vi "Day 13-1.vi"() -> ()   [LabVIEW 2019, in "Day 13.lvlib"]
uses:
  Day 13.lvlib
panel:
  out "size(s)":i32[](array[numeric])
  out "Numeric":i32
  out "Result":bool[][](array[boolean])
  out "Without fold":bool[][](array[boolean])
  out "coordenate":i32[](array[numeric])
  out "axis":string[](array[string])
  out "Points coordenates":i32[][](array[numeric])
  in  "String":string
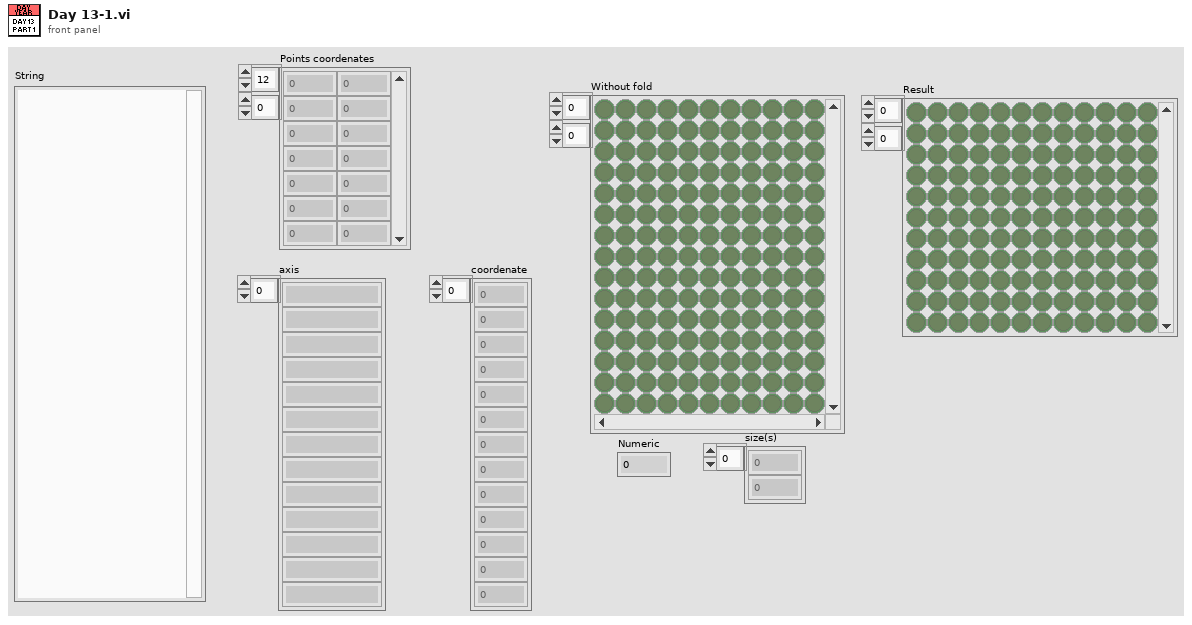
[diagram p1: front panel]
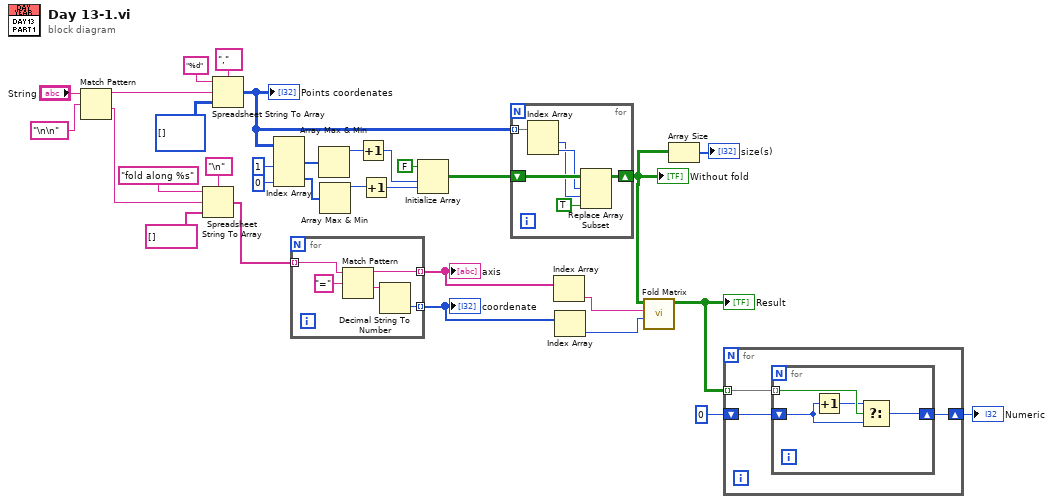
[diagram p0: block diagram]
diagram:
  n1 = Match Pattern(string="String", regular expression="\n\n") -> (before substring=w27:string, after substring=w22:string)  [unwired: 1 in, 2 out]
  n2 = Spreadsheet String To Array(delimiter (Tab)="\n", format string="fold along %s", spreadsheet string=w22, array type (2D Dbl)=string[] []) -> (array=w21:string[])
  n3 = Spreadsheet String To Array(delimiter (Tab)=",", format string="%d", spreadsheet string=w27, array type (2D Dbl)=i32[][] []) -> (array=w19:i32[][])
  "Points coordenates" <- w19
  n4 = Index Array(array=w19, index (col) #1=1 ("disabled index (col)"), index (col) #2=0 ("index (col)")) -> (element #1=w16:i32[], element #2=w15:i32[])  [unwired: 2 in]
  n5 = for {
    tunnel: w21 -> [w36] mode=indexing
    tunnel: [w33] -> w12 mode=indexing
    tunnel: [w32] -> w13 mode=indexing
    n6 = Match Pattern(string=w36, regular expression="=") -> (before substring=w32:string, after substring=w34:string)  [unwired: 1 in, 2 out]
    n7 = Decimal String To Number(string=w34) -> (number=w33:i32)  [unwired: 2 in, 1 out]
  }
  "axis" <- w13
  "coordenate" <- w12
  n8 = Array Max & Min(array=w16) -> (max value=w9:i32)  [unwired: 3 out]
  n9 = Array Max & Min(array=w15) -> (max value=w8:i32)  [unwired: 3 out]
  n10 = Increment(x=w9) -> (x+1=w6:i32)
  n11 = Increment(x=w8) -> (x+1=w7:i32)
  n12 = Initialize Array(FALSE, w6, w7) -> (w14:bool[][])
  n13 = for {
    tunnel: w19 -> [w41] mode=indexing
    shift-right: [w39] -> w2
    shift-left: w14 -> [w42]
    n14 = Index Array(array=w41) -> (element #1=w37:i32, element #2=w38:i32)  [unwired: 2 in]
    n15 = Replace Array Subset(array=w42, new element=TRUE ("new element/subarray"), index (row)=w38, index (col)=w37) -> (w39:bool[][])
  }
  "Without fold" <- w2
  n16 = Index Array(array=w13) -> (element=w11:string)  [unwired: 1 in]
  n17 = Index Array(array=w12) -> (element=w10:i32)  [unwired: 1 in]
  n18 = call "Fold Matrix.vi"("Index"=w10, "Coordenate"=w11, "Dots Matrix"=w2) -> ("Result"=w3:bool[][])  [unwired: 8 in]
  "Result" <- w3
  n19 = Array Size(array=w2) -> (size(s)=→"size(s)":i32[])
  n20 = for {
    tunnel: w3 -> [w45] mode=indexing
    shift-right: [w43] -> w4
    shift-left: 0 -> [w44]
    n21 = for {
      tunnel: w45 -> [w49] mode=indexing
      shift-right: [w46] -> w43
      shift-left: w44 -> [w47]
      n22 = Increment(x=w47) -> (x+1=w48:i32)
      n23 = Select(t=w48, s=w49, f=w47) -> (s? t:f=w46:i32)
    }
  }
  "Numeric" <- w4
